vi "Channel Unload.vi"(8 "error in (no error)":errorcluster, 10 "Channel Index":i32, 11 "Mixer in":refnum<class "Mixer.lvclass">) -> (0 "error out":errorcluster, 3 "Mixer out":refnum<class "Mixer.lvclass">)   [LabVIEW 2020, in "G-Audio.lvlib" / "Mixer.lvclass"]
doc: "Unload the audio data from a channel, and set its state to Empty."
uses:
  Mixer.lvclass
  Mixer.lvclass/Mixer.ctl
  Controls/Message.ctl
  Controls/Command.ctl
  <vilib>/Utility/error.llb/Error Cluster From Error Code.vi
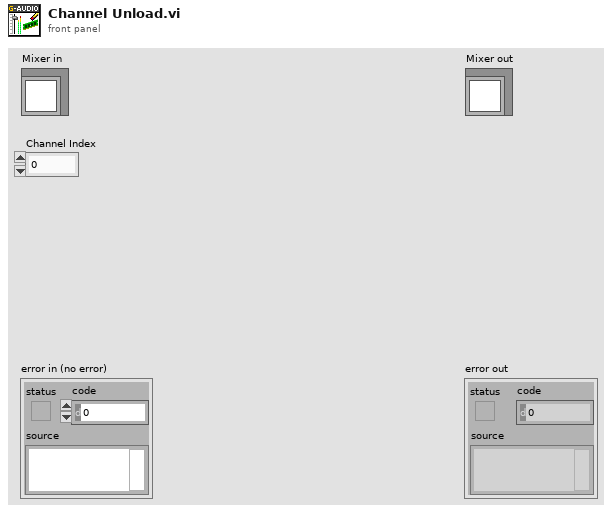
[diagram p1: front panel]
types:
  T1 = typedef "G-Audio.lvlib/Mixer.lvclass/Message.ctl" = cluster{"Command":T2, "Channel":i32, "Payload":variant}
  T2 = typedef "G-Audio.lvlib/Mixer.lvclass/Command.ctl" = enum16{"Channel Stop", "Channel Pause", "Channel Play", "Channel Volume", "Channel Unload"}
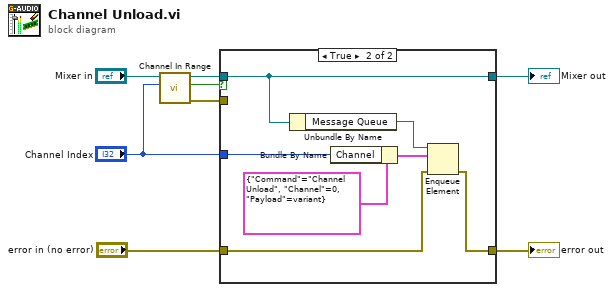
[diagram p0: block diagram]
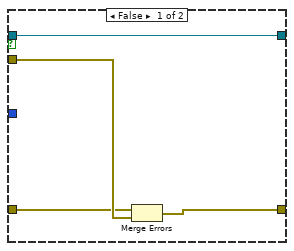
[diagram p2: hidden frame]
diagram:
  n1 = call "Channel In Range.vi"("Channel Index"="Channel Index", "Mixer in"="Mixer in") -> ("error out"=w4:errorcluster, "In Range"=w6:bool, "Mixer out"=w7:refnum<class "Mixer.lvclass">)  [unwired: 7 in]
  n2 = case shown="True" w6 {
    tunnel: w7 -> [w12 w13]
    tunnel: "Channel Index" -> [_ w16]
    tunnel: "error in (no error)" -> [w10 w15]
    tunnel: [w9 w14] -> w2
    tunnel: [w12 w13] -> w1
    tunnel: w4 -> [w11 _]
    frame False {
      n3 = Merge Errors(w10, w11) -> (w9:errorcluster)
    }
    frame True {
      n4 = Unbundle By Name(w13) -> ("Message Queue"=w19:refnum<queue>)
      n5 = Bundle By Name(cluster=T1 {"Command"=enum."Channel Unload", "Channel"=0, "Payload"=variant} ("element"), "Channel"=w16) -> (w17:T1)
      n6 = Enqueue Element(queue=w19, element=w17, error in (no error)=w15) -> (error out=w14:errorcluster)  [unwired: 1 in, 2 out]
    }
  }
  "error out" <- w2
  "Mixer out" <- w1
